vi "Geomatric ]PatternMatch_MainFunction.vi"(0 "Geomatric Match Parameter":T2={"Curve Extraction"={"Extraction Mode"=0, "Edge Threshold"=75, "Edge Filter Size"=1, "Min Length"=25, "Row Search Step Size"=15, "Column Search Step Size"=15, "Max Endpoint Gap"=10, "Closed"=FALSE, "Subpixel"=FALSE}, "X Position Offset"=0, "Y Position Offset"=0, "Match Parameters"={"Number of Matches Requested"=1, "Minimum Match Score"=750.0, "Angle Ranges"=[]}, "Template path"="", "Range Settings"=[], "Match Mode"={"Rotation"=TRUE, "Scale"=FALSE, "Occlusion"=FALSE, "Reserved"=FALSE, "Reserved"=FALSE, "Reserved"=FALSE}} {"Range Settings"."Match Constraints" items=["Rotation Angle (degrees)", "Scale Factor (%)", "Occlusion (%)"]; "Match Parameters"."Angle Ranges"."End Angle" min=-360 max=360; "Match Parameters"."Angle Ranges"."Start Angle" min=-360 max=360; "Match Parameters"."Minimum Match Score" min=0 max=1000; "Match Parameters"."Number of Matches Requested" min=1 max=9999; "Curve Extraction"."Edge Filter Size" items=["Fine", "Normal", "Contour Tracing"]; "Curve Extraction"."Edge Threshold" min=0 max=255 step=1; "Curve Extraction"."Extraction Mode" items=["Normal", "Uniform Regions"]}, 5 "Vision_Image In":T4, 9 "ROI Descriptor":T5 {"Contours"."Type" items=["No Selection", "Point", "Line", "Rectangle", "Oval", "Polygon", "Freehand Region", "Annulus", "Unused2", "Unused3", "Broken Line", "Freehand Line", "Rotated Rectangle"]}, 11 "error in":errorcluster) -> (4 "Matches (pixel)":T1[](array[typedef]) {"Correlation Score" format="%.2f"; "Target Template Curve Score" format="%.2f"; "Template Target Curve Score" format="%.2f"; "Bounding Box"."y" format="%.2f"; "Bounding Box"."x" format="%.2f"; "Position"."y" format="%.2f"; "Position"."x" format="%.2f"; "Score" format="%.2f"; "Scale" format="%.2f"; "Angle" format="%.2f"; "Occlusion %" format="%.2f"}, 6 "Matches (real-world)":T1[](array[typedef]) {"Correlation Score" format="%.2f"; "Target Template Curve Score" format="%.2f"; "Template Target Curve Score" format="%.2f"; "Bounding Box"."y" format="%.2f"; "Bounding Box"."x" format="%.2f"; "Position"."y" format="%.2f"; "Position"."x" format="%.2f"; "Score" format="%.2f"; "Scale" format="%.2f"; "Angle" format="%.2f"; "Occlusion %" format="%.2f"}, 8 "Image (duplicate)":T4(plugin-control), 10 "Number of Matches":i32, 15 "error out":errorcluster)   [LabVIEW 2019]
uses:
  <vilib>/vision/Image Controls.llb/IMAQ Image.ctl
  Controls/Geometric Match/Analysis_Geometric PatternMatch_Parameter.ctl
  <vilib>/vision/Pattern Matching.llb/IMAQ Match Range Setting.ctl
  <vilib>/vision/Pattern Matching.llb/IMAQ GM Match Report.ctl
  <vilib>/vision/NI_Vision_Development_Module.lvlib
panel:
  out "Image":T4(plugin-control)
  out "Template In":T4
  # "Range"
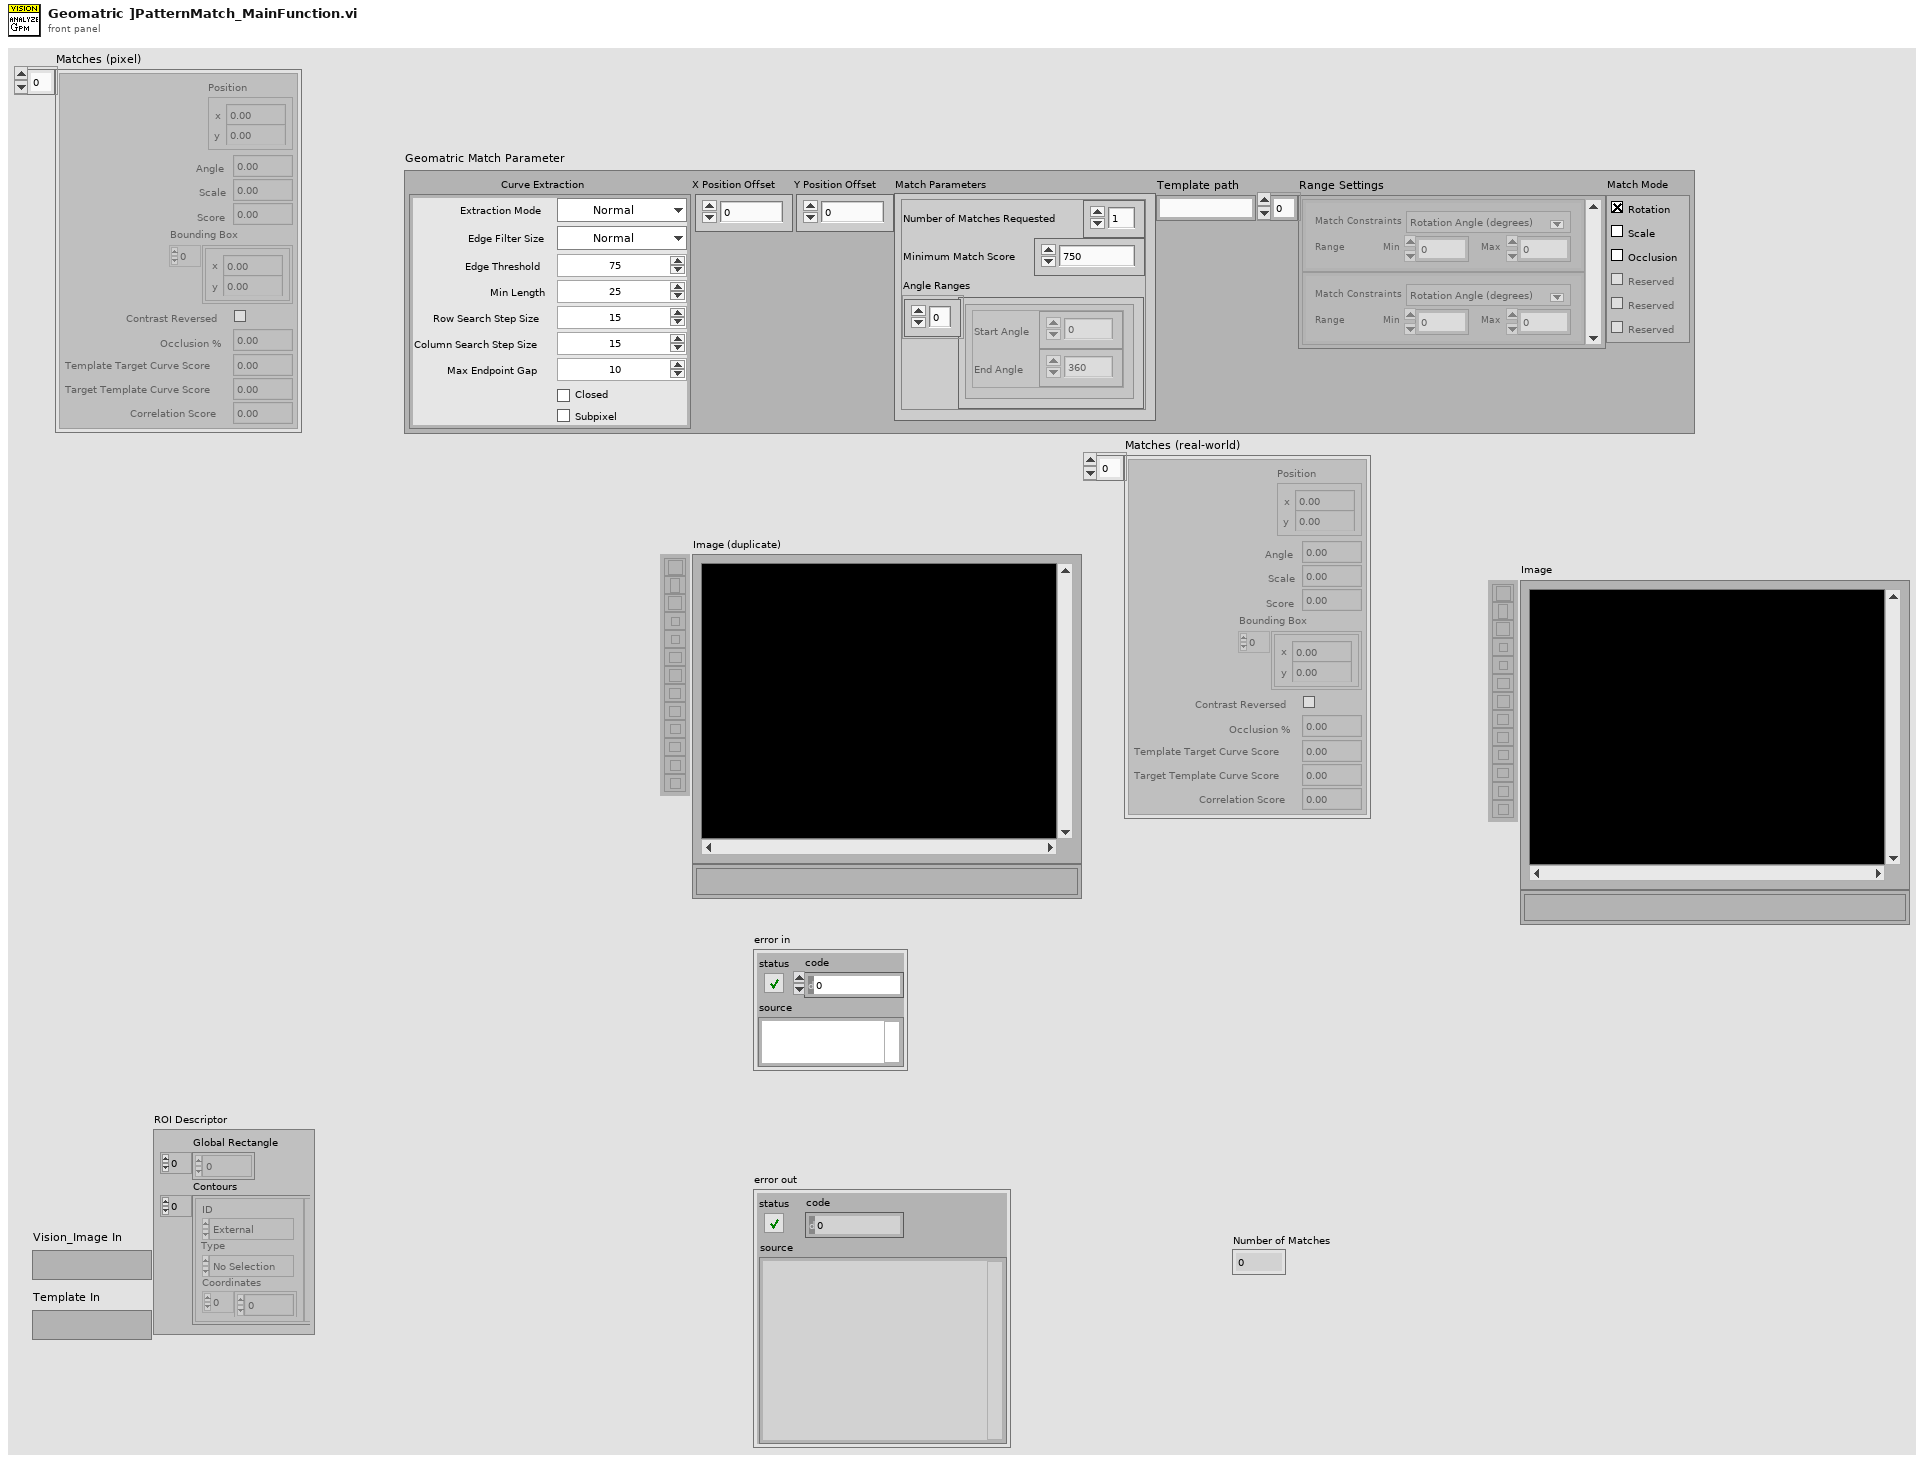
[diagram p1: front panel]
types:
  T1 = typedef "IMAQ GM Match Report.ctl" = cluster{"Position":cluster{"x":sgl, "y":sgl}, "Angle":sgl, "Scale":sgl, "Score":sgl, "Bounding Box":cluster{"x":sgl, "y":sgl}[], "Contrast Reversed":bool, "Occlusion %":sgl, "Template Target Curve Score":sgl, "Target Template Curve Score":sgl, "Correlation Score":sgl}
  T2 = typedef "Analysis_Geometric PatternMatch_Parameter.ctl" = cluster{"Curve Extraction":cluster{"Extraction Mode":u32, "Edge Threshold":i32, "Edge Filter Size":u32, "Min Length":i32, "Row Search Step Size":i32, "Column Search Step Size":i32, "Max Endpoint Gap":i32, "Closed":bool, "Subpixel":bool}, "X Position Offset":i32, "Y Position Offset":i32, "Match Parameters":cluster{"Number of Matches Requested":i32, "Minimum Match Score":sgl, "Angle Ranges":cluster{"Start Angle":sgl, "End Angle":sgl}[]}, "Template path":string, "Range Settings":T3[], "Match Mode":cluster{"Rotation":bool, "Scale":bool, "Occlusion":bool, "Reserved":bool, "Reserved":bool, "Reserved":bool}}
  T3 = typedef "IMAQ Match Range Setting.ctl" = cluster{"Match Constraints":u32, "Min":dbl, "Max":dbl}
  T4 = typedef "IMAQ Image.ctl" = refnum<image>
  T5 = typedef "ROI Descriptor" = cluster{"Global Rectangle":i32[], "Contours":cluster{"ID":enum32{"External", "Internal"}, "Type":u32, "Coordinates":i32[]}[]}
  T6 = cluster{"Extraction Mode":u32, "Edge Threshold":i32, "Edge Filter Size":u32, "Min Length":i32, "Row Search Step Size":i32, "Column Search Step Size":i32, "Max Endpoint Gap":i32, "Closed":bool, "Subpixel":bool}
  T7 = cluster{"Number of Matches Requested":i32, "Minimum Match Score":sgl, "Angle Ranges":cluster{"Start Angle":sgl, "End Angle":sgl}[]}
  T8 = cluster{"Rotation":bool, "Scale":bool, "Occlusion":bool, "Reserved":bool, "Reserved":bool, "Reserved":bool}
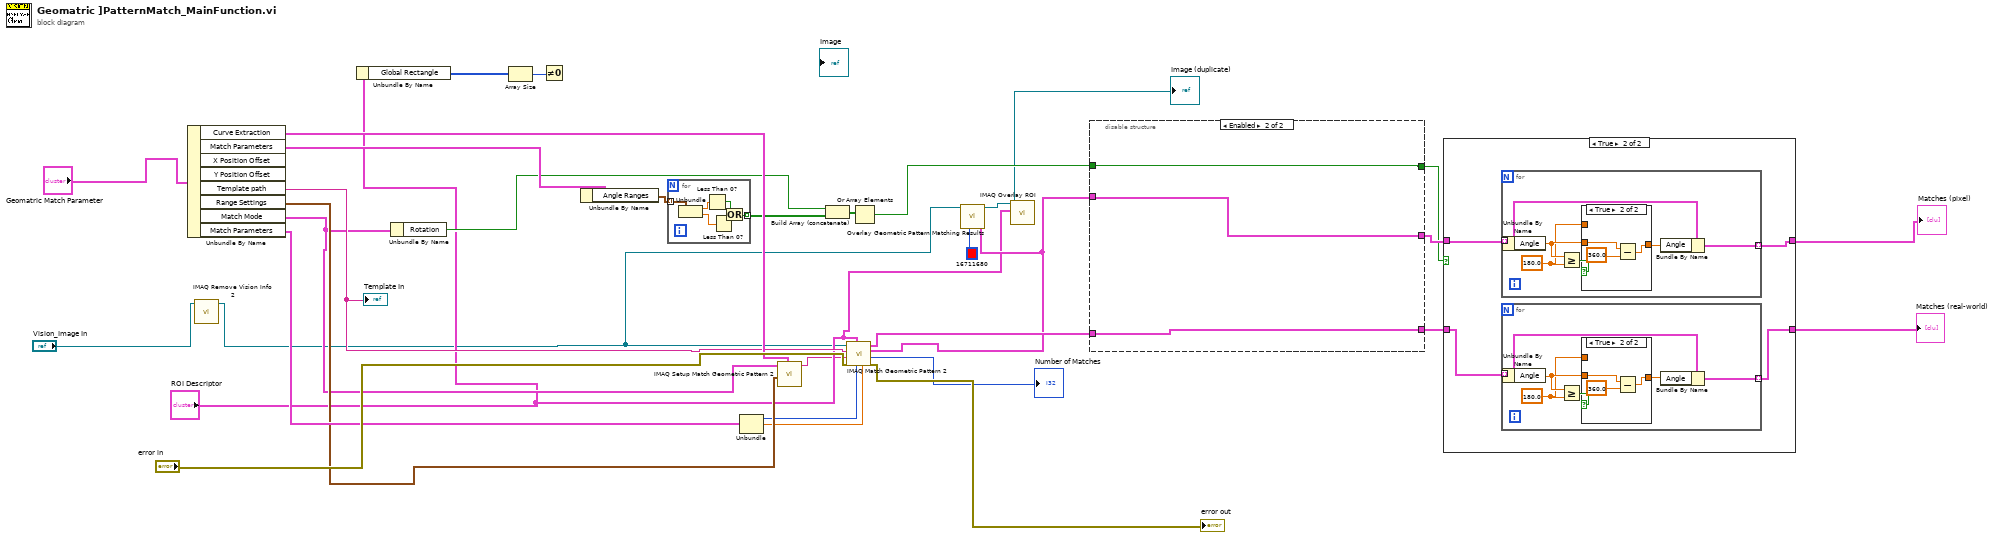
[diagram p0: block diagram]
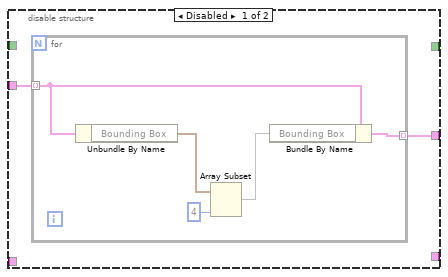
[diagram p5: hidden frame]
diagram:
  n1 = Unbundle By Name("Geomatric Match Parameter") -> ("Curve Extraction"=w29:T6, "Match Parameters"=w27:T7, "Template path"=w20:string, "Range Settings"=w11:T3[], "Match Mode"=w10:T8, "Match Parameters"=w18:T7)  [unwired: 2 out]
  "Template In" <- w20
  n2 = call "IMAQ Remove Vision Info 2"("Image"="Vision_Image In") -> ("Image Out"=w1:T4)  [unwired: 9 in, 1 out]
  n3 = Unbundle By Name("ROI Descriptor") -> ("Global Rectangle"=w30:i32[])
  n4 = Unbundle By Name(w10) -> ("Rotation"=w9:bool)
  n5 = Array Size(array=w30) -> (size(s)=w31:i32)
  n6 = Not Equal To 0?(x=w31) -> ()  [unwired: 1 out]
  n7 = Unbundle By Name(w27) -> ("Angle Ranges"=w21:cluster{"Start Angle":sgl, "End Angle":sgl}[])
  n8 = for {
    tunnel: w21 -> [w39] mode=indexing
    tunnel: [w34] -> w26 mode=indexing
    n9 = Unbundle(w39) -> ("Start Angle"=w38:sgl, "End Angle"=w37:sgl)
    n10 = Less Than 0?(x=w38) -> (x < 0?=w36:bool)
    n11 = Less Than 0?(x=w37) -> (x < 0?=w35:bool)
    n12 = Or(x=w36, y=w35) -> (x .or. y?=w34:bool)
  }
  n13 = Unbundle(w18) -> ("Number of Matches Requested"=w4:i32, "Minimum Match Score"=w3:sgl)  [unwired: 1 out]
  n14 = call "IMAQ Setup Match Geometric Pattern 2"("Curve Parameters"=w29, "Range Settings"=w11, "Match Mode"=w10) -> ("Match Geometric Pattern 2 Setup Data"=w5:string)  [unwired: 7 in, 1 out]
  n15 = Build Array (concatenate)(w9, w26) -> (w12:bool[])
  n16 = call "IMAQ Match Geometric Pattern 2"("Minimum Match Score"=w3, "Number of Matches Requested"=w4, "ROI Descriptor"="ROI Descriptor", "error in (no error)"="error in", "Match Geometric Pattern 2 Setup Data"=w5, "Template Image"=w20, "Image"=w1) -> ("error out"=→"error out":errorcluster, "Number of Matches"=→"Number of Matches":i32, "Matches (real-world)"=w7:T1[], "Matches (pixel)"=w28:T1[])  [unwired: 1 in]
  n17 = Or Array Elements(Boolean array=w12) -> (logical OR=w22:bool)
  n18 = call "Overlay Geometric Pattern Matching Results.vi"("Color"=u32 16711680, "Matches"=w7, "Image"=w1) -> ("Image Out"=w14:T4)  [unwired: 7 in, 1 out]
  n19 = call "IMAQ Overlay ROI"("ROI Descriptor"="ROI Descriptor", "Image"=w14) -> ("Image Out"=→"Image (duplicate)":T4)  [unwired: 8 in, 1 out]
  n20 = disable-structure shown="Enabled" {
    disable-tunnel: w7 -> [w41 w49]
    disable-tunnel: [w40 w49] -> w25
    disable-tunnel: w28 -> [_ w48]
    disable-tunnel: [_ w48] -> w24
    disable-tunnel: [_ w47] -> w23
    disable-tunnel: w22 -> [_ w47]
    frame Disabled {
      n21 = for {
        tunnel: w41 -> [w45] mode=indexing
        tunnel: [w42] -> w40 mode=indexing
        n22 = Unbundle By Name(w45) -> ("Bounding Box"=w44:cluster{"x":sgl, "y":sgl}[])
        n23 = Array Subset(array=w44, length=4) -> (w43:cluster{"x":sgl, "y":sgl}[])  [unwired: 1 in]
        n24 = Bundle By Name(cluster=w45, "Bounding Box"=w43) -> (w42:T1)
      }
    }
    frame Enabled {
    }
  }
  n25 = case shown="True" w23 {
    tunnel: [w51 w54] -> w16
    tunnel: w25 -> [w51 w55]
    tunnel: [w50 w52] -> w15
    tunnel: w24 -> [w50 w53]
    frame False {
    }
    frame True {
      n26 = for {
        tunnel: w55 -> [w68] mode=indexing
        tunnel: [w66] -> w54 mode=indexing
        w69 = sgl 180.0 ("y")
        n27 = Unbundle By Name(w68) -> ("Angle"=w70:sgl)
        n28 = Greater Or Equal?(x=w70, y=w69) -> (x >= y?=w71:bool)
        n29 = case shown="True" w71 {
          tunnel: w70 -> [w72 w74]
          tunnel: w69 -> [_ _]
          tunnel: [w72 w75] -> w67
          frame False {
          }
          frame True {
            n30 = Subtract(x=w74, y=sgl 360.0) -> (x-y=w75:sgl)
          }
        }
        n31 = Bundle By Name(cluster=w68, "Angle"=w67) -> (w66:T1)
      }
      n32 = for {
        tunnel: w53 -> [w58] mode=indexing
        tunnel: [w56] -> w52 mode=indexing
        w59 = sgl 180.0 ("y")
        n33 = Unbundle By Name(w58) -> ("Angle"=w60:sgl)
        n34 = Greater Or Equal?(x=w60, y=w59) -> (x >= y?=w61:bool)
        n35 = case shown="True" w61 {
          tunnel: w60 -> [w62 w64]
          tunnel: w59 -> [_ _]
          tunnel: [w62 w65] -> w57
          frame False {
          }
          frame True {
            n36 = Subtract(x=w64, y=sgl 360.0) -> (x-y=w65:sgl)
          }
        }
        n37 = Bundle By Name(cluster=w58, "Angle"=w57) -> (w56:T1)
      }
    }
  }
  "Matches (pixel)" <- w16
  "Matches (real-world)" <- w15
